vi "Multiply.vi"   [LabVIEW 2017, in "NI_Matrix.lvlib"]
doc: "Returns the product of the inputs."
uses:
  <vilib>/Analysis/Matrix/NI_Matrix.lvlib
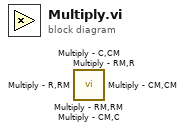
[diagram p0: block diagram]
diagram:
  n1 = call <vilib>:"Multiply - RM,RM.vi"() -> ()  [unwired: 2 in, 1 out]
  n2 = call <vilib>:"Multiply - RM,R.vi"() -> ()  [unwired: 2 in, 1 out]
  n3 = call <vilib>:"Multiply - R,RM.vi"() -> ()  [unwired: 2 in, 1 out]
  n4 = call <vilib>:"Multiply - CM,CM.vi"() -> ()  [unwired: 2 in, 1 out]
  n5 = call <vilib>:"Multiply - CM,C.vi"() -> ()  [unwired: 2 in, 1 out]
  n6 = call <vilib>:"Multiply - C,CM.vi"() -> ()  [unwired: 2 in, 1 out]
